vi "Simulated_Amperometer.vi"(8 "error in (no error)":errorcluster, 11 "Device Name":tag) -> (0 "error out":errorcluster, 3 "Measurement":dbl)   [LabVIEW 2023]
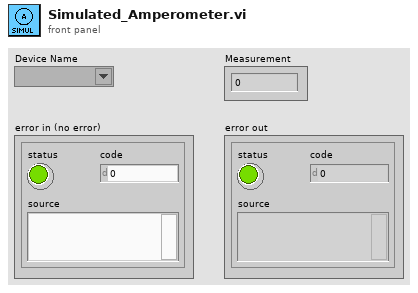
[diagram p1: front panel]
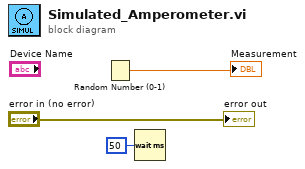
[diagram p0: block diagram]
diagram:
  n1 = Random Number (0-1)() -> (number: 0 to 1=→"Measurement":dbl)
  n2 = Wait (ms)(milliseconds to wait=u32 50) -> ()  [unwired: 1 out]
  "error out" <- "error in (no error)"
